vi "initialize task components.vi"(7 "ID":string, 9 "task token":refnum<class "null task token.lvclass">, 10 "results reporter":refnum<class "results reporter.lvclass">, 11 "task in":refnum<class "task.lvclass">) -> (3 "task out":refnum<class "task.lvclass">)   [LabVIEW 2013, in "task.lvclass"]
uses:
  task.lvclass
  task token/null task token.lvclass
  results reporter/results reporter.lvclass
  task.lvclass/task.ctl
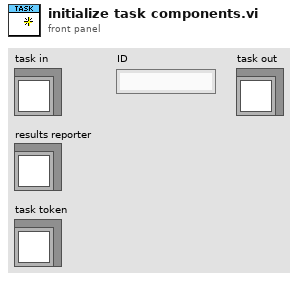
[diagram p1: front panel]
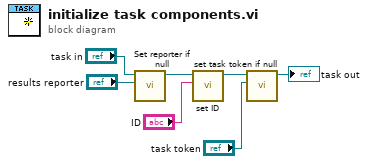
[diagram p0: block diagram]
diagram:
  n1 = call "Set reporter if null.vi"("results reporter"="results reporter", "task in"="task in") -> ("task out"=w7:refnum<class "task.lvclass">)  [unwired: 9 in]
  n2 = call "set ID.vi"("ID"="ID", "task in"=w7) -> ("task out"=w6:refnum<class "task.lvclass">)  [unwired: 9 in]
  n3 = call "set task token if null.vi"("task token"="task token", "task in"=w6) -> ("task out"=→"task out":refnum<class "task.lvclass">)  [unwired: 9 in]
